vi "tdms_open.vi"() -> ()   [LabVIEW 2019]
panel:
  out "error out":errorcluster
  out "property values":variant[](array[variant])
  out "channel name(s) out":string[](array[string])
  out "group name out":string
  out "Waveform Graph":waveform(dbl)[](graph)
  in  "file path":path
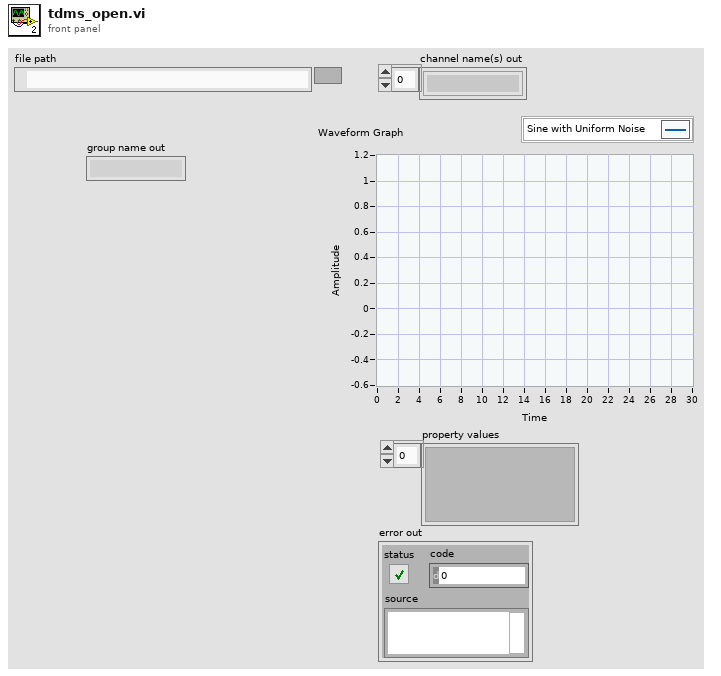
[diagram p1: front panel]
types:
  T1 = enum16{"big-endian, network order", "native, host order", "little-endian"}
  T2 = enum16{"open", "open or create", "create or replace", "create", "open (read-only)"}
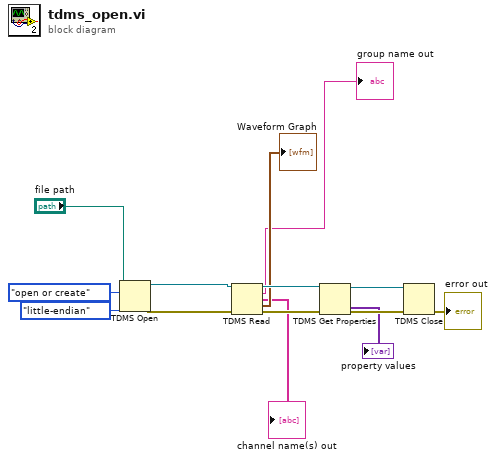
[diagram p0: block diagram]
diagram:
  n1 = TDMS Open(9:T1."little-endian" ("byte order (2:little-endian)"), 10:T2."open or create" ("operation (0:open)"), 11:"file path") -> (0:w13:errorcluster, 3:w14:refnum<k34>)  [unwired: 4 in]
  n2 = TDMS Read(0:w14, 11:w13) -> (4:w12:refnum<k34>, 6:→"group name out":string, 8:→"channel name(s) out":string[], 10:→"Waveform Graph":waveform(dbl)[], 15:w9:errorcluster)  [unwired: 6 in, 1 out]
  n3 = TDMS Get Properties(8:w9, 11:w12) -> (0:w10:errorcluster, 3:w11:refnum<k34>, 4:→"property values":variant[])  [unwired: 4 in, 3 out]
  n4 = TDMS Close(8:w10, 11:w11) -> (0:→"error out":errorcluster)  [unwired: 1 out]
